vi "FA_MultiReadETag.vi"(6 "Error In":errorcluster, 8 "ID Array":string[](array[string])) -> (0 "Error Out":errorcluster, 1 "ETagArray":string[](array[string]))   [LabVIEW 2014, in "FA_LocalStore.lvlib"]
doc: "Given an array of Special Type this VI returns an array of that special type's eTag in LocalStore"
uses:
  FA_LocalStore.lvlib
  <vilib>/Utility/config.llb/Read Key (String).vi
  <vilib>/Utility/config.llb/NI_LVConfig.lvlib
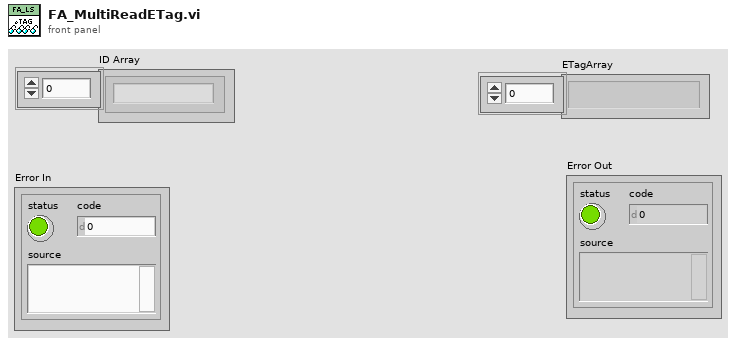
[diagram p1: front panel]
types:
  T1 = typedef "FA_LocalStore.lvlib/FA_LSRef.ctl" = cluster{"eTag INI Refnum":T2, "XML Refnum Array":refnum<file>[]}
  T2 = typedef "NI_LVConfig.lvlib/Config Data RefNum.ctl" = refnum<k1>
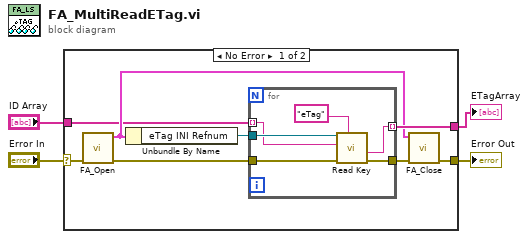
[diagram p0: block diagram]
diagram:
  n1 = case shown="No Error" "Error In" {
    selector: "Error In" -> [w8 w19]
    tunnel: [w9 w19] -> w3
    tunnel: "ID Array" -> [w6 _]
    tunnel: [w11 _] -> w1
    frame No Error {
      n2 = call "FA_Open.vi"("Error In"=w8) -> ("Error Out"=w5:errorcluster, "FA_LS Ref"=w7:T1)  [unwired: 9 in]
      n3 = Unbundle By Name(w7) -> ("eTag INI Refnum"=w12:T2)
      n4 = for {
        tunnel: w12 -> [w17]
        tunnel: [w16] -> w11 mode=indexing
        tunnel: [w15] -> w10
        tunnel: w6 -> [w14] mode=indexing
        tunnel: w5 -> [w13]
        n5 = call-poly <vilib>:"Read Key.vi"("section"="eTag", "error in (no error)"=w13, "key"=w14, "refnum"=w17) -> ("error out"=w15:errorcluster, "value"=w16:string)  [unwired: 4 in, 2 out]
      }
      n6 = call "FA_Close.vi"("Error In"=w10, "FA_LS Ref"=w7) -> ("Error Out"=w9:errorcluster)  [unwired: 9 in]
    }
    frame Error {
    }
  }
  "Error Out" <- w3
  "ETagArray" <- w1
